vi "Send_start.vi"(8 "error in":errorcluster) -> (0 "error out":errorcluster)   [LabVIEW 2018]
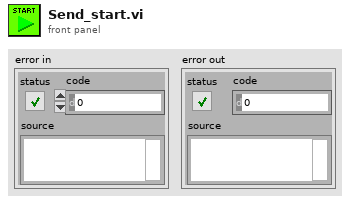
[diagram p1: front panel]
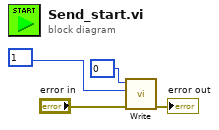
[diagram p0: block diagram]
diagram:
  n1 = call "Write.vi"("error in"="error in", "Data to write"=u8 1 ("Slave Address (7-bit)"), "Address"=u8 0 ("Slave Address (7-bit)")) -> ("error out"=→"error out":errorcluster)  [unwired: 8 in]
